vi "POST-Multipart.vi"(6 "timeout":i32=10000, 7 "output file":path, 8 "error in":errorcluster, 9 "Multipart Post data":T1[](array[typedef]), 10 "url":string, 11 "http-client in":refnum<class "http-client.lvclass">) -> (0 "error out":errorcluster, 1 "body":string, 2 "headers":string, 3 "http-client out":refnum<class "http-client.lvclass">, 4 "status code":u16)   [LabVIEW 2025, in "http-client.lvclass"]
uses:
  http-client.lvclass
  <vilib>/httpClient/MultipartData.ctl
  <vilib>/httpClient/LabVIEWHTTPClient.lvlib
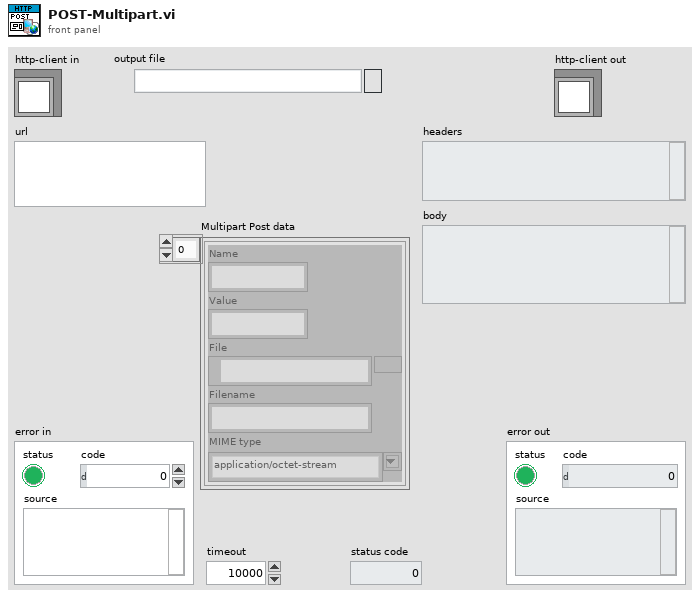
[diagram p1: front panel]
types:
  T1 = typedef "LabVIEWHTTPClient.lvlib/MultipartData.ctl" = cluster{"Name":string, "Value":string, "File":path, "Filename":string, "MIME type":string}
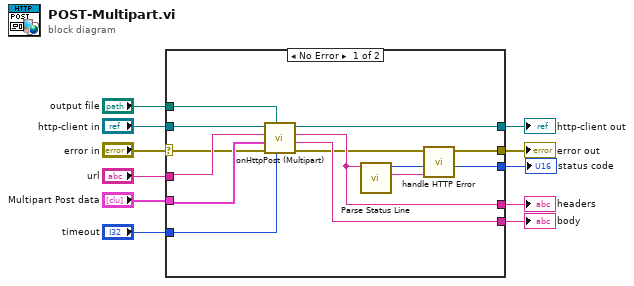
[diagram p0: block diagram]
diagram:
  n1 = case shown="No Error" "error in" {
    selector: "error in" -> [w21 w27]
    tunnel: [w15 w27] -> w10
    tunnel: [w20 w26] -> w8
    tunnel: "http-client in" -> [w25 w26]
    tunnel: [w17 _] -> w7
    tunnel: "url" -> [w22 _]
    tunnel: "timeout" -> [w24 _]
    tunnel: "output file" -> [w19 _]
    tunnel: [w18 _] -> w3
    tunnel: "Multipart Post data" -> [w23 _]
    tunnel: [w12 _] -> w1
    frame No Error {
      n2 = call-dynamic "onHttpPost (Multipart).vi"("timeout"=w24, "output file"=w19, "error in"=w21, "Multipart Post data"=w23, "url"=w22, "http-method in"=w25) -> ("error out"=w16:errorcluster, "body"=w18:string, "headers"=w17:string, "http-method out"=w20:refnum<class "http-client.lvclass">)  [unwired: 2 in]
      n3 = call "Parse Status Line.vi"("Headers w/ status line"=w17) -> ("Status String"=w13:string, "status code"=w14:u16)  [unwired: 6 in, 3 out]
      n4 = call "handle HTTP Error.vi"("Status String"=w13, "status code"=w14, "error in (no error)"=w16) -> ("status code dup"=w12:u16, "error out"=w15:errorcluster)  [unwired: 7 in]
    }
    frame Error {
    }
  }
  "error out" <- w10
  "http-client out" <- w8
  "headers" <- w7
  "body" <- w3
  "status code" <- w1
